vi "Motor_Ctrl.vi"(7 "Reset":bool, 8 "error in (no error)":errorcluster, 9 "TargetRPM(+/-120)":dbl format="%.2f", 10 "B/BL Motor":T1 items=["BLDC", "BDC"], 11 "Port":T2) -> (0 "error out":errorcluster, 1 "RPM/T Chart":cluster{"upper limit":dbl, "RPM":dbl}(graph), 2 "Rotations":dbl, 3 "RPM":dbl)   [LabVIEW 2019, in "Motor_Lib.lvlib"]
uses:
  Motor_Lib.lvlib
  PORT_ID.ctl
  MotorType.ctl
  <vilib>/myRIO/Instrument Drivers/Onboard IO/AO/typedefs/AO Reference.ctl
  <vilib>/myRIO/Common/Instrument Driver Framework/Utilities/typedefs/myRIO Generic Hardware Reference.ctl
  <vilib>/myRIO/Common/Instrument Driver Framework/Utilities/typedefs/Hardware Version Enum.ctl
  <vilib>/myRIO/Common/Instrument Driver Framework/Utilities/typedefs/myRIO v1.0 Reference.ctl
  <vilib>/myRIO/Common/Instrument Driver Framework/Utilities/typedefs/Generic FPGA Reference.ctl
  <vilib>/myRIO/Common/Instrument Driver Framework/myRIO v1.0/AO/typedefs/AO Channels List.ctl
  <vilib>/myRIO/Common/Instrument Driver Framework/myRIO v1.0/AO/typedefs/AO Channels Enum.ctl
  <vilib>/myRIO/Common/Instrument Driver Framework/Utilities/typedefs/Analog Scaling Constants List.ctl
  <vilib>/myRIO/Common/Instrument Driver Framework/Utilities/typedefs/Analog Scaling Constants.ctl
  <vilib>/userDefined/High Color/nirio_resource_hc.ctl
  <vilib>/myRIO/Instrument Drivers/Onboard IO/PWM/typedefs/PWM Reference.ctl
  <vilib>/myRIO/Common/Instrument Driver Framework/myRIO v1.0/PWM/typedefs/PWM Channels Enum.ctl
  <vilib>/myRIO/Instrument Drivers/Onboard IO/PWM/typedefs/PWM Configuration.ctl
  <vilib>/myRIO/Instrument Drivers/Onboard IO/DIO/typedefs/DIO Reference.ctl
  <vilib>/myRIO/Common/Instrument Driver Framework/myRIO v1.0/DIO/typedefs/DIO Channels List.ctl
  <vilib>/myRIO/Common/Instrument Driver Framework/myRIO v1.0/DIO/typedefs/DIO Channels Enum.ctl
  <vilib>/myRIO/Instrument Drivers/Onboard IO/PWM/vis/Set Duty Cycle and Frequency.vi
  <vilib>/myRIO/Common/Instrument Driver Framework/myRIO v1.0/PWM/vis/myRIO v1.1 Open PWM.vi
  <vilib>/myRIO/Common/Instrument Driver Framework/Utilities/vis/Is FPGA Ref Available.vi
  <vilib>/myRIO/Instrument Drivers/Onboard IO/DIO/vis/Write.vi
  <vilib>/myRIO/Common/Instrument Driver Framework/myRIO v1.0/DIO/vis/myRIO v1.1 Open DIO.vi
  <vilib>/myRIO/Instrument Drivers/Onboard IO/AO/vis/Write.vi
  <vilib>/myRIO/Common/Instrument Driver Framework/myRIO v1.0/AO/vis/myRIO v1.1 Open AO.vi
  <vilib>/myRIO/Common/Instrument Driver Framework/Utilities/vis/Validate Channels.vi
  <vilib>/myRIO/Common/Instrument Driver Framework/myRIO v1.0/PWM/vis/myRIO v1.0 Reserve PWM.vi
  <vilib>/myRIO/Common/Instrument Driver Framework/myRIO v1.0/DIO/vis/myRIO v1.0 Reserve DIO.vi
  <vilib>/myRIO/Common/Instrument Driver Framework/myRIO v1.0/AO/vis/myRIO v1.0 Reserve AO.vi
  <vilib>/myRIO/Common/Instrument Driver Framework/myRIO v1.0/PWM/vis/myRIO v1.0 Build MUX Configuration PWM.vi
  <vilib>/myRIO/Common/Instrument Driver Framework/myRIO v1.0/Resource Manager/vis/myRIO v1.0 Reserve Channel List.vi
  <vilib>/myRIO/Common/Instrument Driver Framework/myRIO v1.0/DIO/vis/myRIO v1.0 Build MUX Configuration DIO.vi
  <vilib>/myRIO/Common/Instrument Driver Framework/myRIO v1.0/AO/vis/myRIO v1.0 Build MUX Configuration AO.vi
  <vilib>/myRIO/Common/Instrument Driver Framework/myRIO v1.0/Resource Manager/vis/myRIO v1.0 Create Configuration List.vi
  <vilib>/myRIO/Common/Instrument Driver Framework/myRIO v1.0/Resource Manager/vis/myRIO v1.0 Reserve Channel.vi
  <vilib>/myRIO/Common/Instrument Driver Framework/myRIO v1.0/Resource Manager/vis/myRIO v1.0 Unreserve Channel.vi
  <vilib>/myRIO/Common/Instrument Driver Framework/myRIO v1.0/Resource Manager/vis/myRIO v1.0 Build Mutex Name.vi
  <vilib>/addons/control/pid/pid.llb/PID (DBL).vi
  <vilib>/Utility/VariantDataType/GetNumericInfo.vi
  <vilib>/Utility/error.llb/Error Cluster From Error Code.vi
  <vilib>/myRIO/Common/Instrument Driver Framework/myRIO v1.0/myRIO v1.1 Open.vi
  <vilib>/myRIO/Common/Instrument Driver Framework/myRIO v1.0/AO/vis/myRIO v1.0 Get Scaling Constants AO.vi
  <vilib>/myRIO/Common/Instrument Driver Framework/Utilities/vis/IO Manager.vi
  <vilib>/myRIO/Common/Instrument Driver Framework/Utilities/vis/Configuration Manager.vi
  <vilib>/myRIO/Common/Instrument Driver Framework/myRIO v1.0/myRIO v1.0 Close.vi
  <vilib>/myRIO/Common/Instrument Driver Framework/myRIO v1.0/AO/vis/myRIO v1.0 Write AO.vi
  <vilib>/myRIO/Common/Instrument Driver Framework/myRIO v1.0/Resource Manager/vis/myRIO v1.0 Configure IO.vi
  <vilib>/myRIO/Common/Instrument Driver Framework/myRIO v1.0/DIO/vis/myRIO v1.0 Write DIO.vi
  <vilib>/myRIO/Common/Instrument Driver Framework/myRIO v1.0/PWM/vis/myRIO v1.0 Write PWM.vi
  <vilib>/myRIO/Express VI/Onboard IO/AO/AO Express VI.xnode
  <vilib>/myRIO/Instrument Drivers/Onboard IO/AO/vis/myRIO AO Open.xnode
  <vilib>/myRIO/Express VI/Onboard IO/DO/DO Express VI.xnode
  <vilib>/myRIO/Instrument Drivers/Onboard IO/DIO/vis/myRIO DIO Open.xnode
  <vilib>/myRIO/Express VI/Onboard IO/PWM/PWM Express VI.xnode
  <vilib>/myRIO/Instrument Drivers/Onboard IO/PWM/vis/myRIO PWM Open.xnode
  <vilib>/myRIO/Instrument Drivers/Onboard IO/PWM/PWM.lvlib
  <vilib>/addons/control/pid/NI_PID_pid.lvlib
  <vilib>/myRIO/Instrument Drivers/Onboard IO/DIO/DIO.lvlib
  <vilib>/myRIO/Instrument Drivers/Onboard IO/AO/AO.lvlib
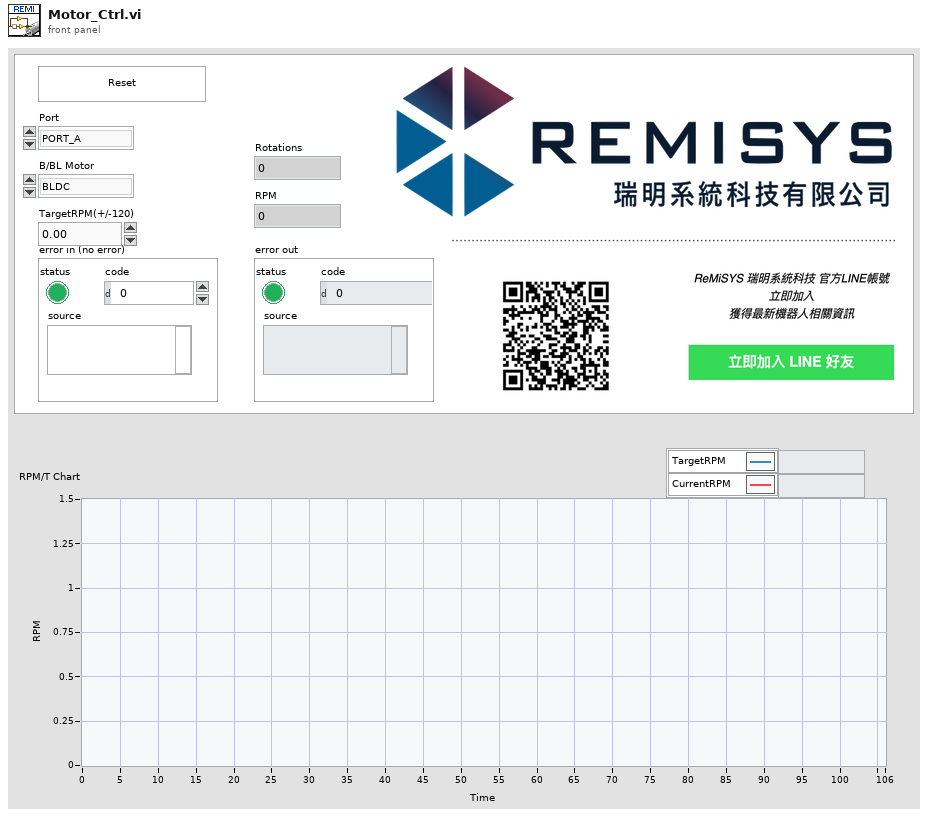
[diagram p1: front panel]
types:
  T1 = typedef "Motor_Lib.lvlib/MotorType.ctl" = u16
  T2 = typedef "Motor_Lib.lvlib/PORT_ID.ctl" = enum16{"PORT_A", "PORT_B"}
  T3 = cluster{"proportional gain (Kc)":dbl, "integral time (Ti, min)":dbl, "derivative time (Td, min)":dbl}
  T4 = typedef "AO.lvlib/AO Reference.ctl" = cluster{"myRIO Reference":T5, "AO Channel List":T9, "AO Scaling Constant List":T11}
  T5 = typedef "myRIO Generic Hardware Reference.ctl" = cluster{"myRIO Model":T6, "myRIO Hardware Reference":T7}
  T6 = typedef "Hardware Version Enum.ctl" = enum16{"Unknown", "myRIO-1900", "myRIO-1950", "roboRIO", "NI ELVIS RIO CM", "ELVIS III"}
  T7 = typedef "myRIO v1.0 Reference.ctl" = cluster{"Generic FPGA Reference":T8, "Allow multiple opens":bool}
  T8 = typedef "Generic FPGA Reference.ctl" = refnum<k20>
  T9 = typedef "AO Channels List.ctl" = T10[]
  T10 = typedef "AO Channels Enum.ctl" = enum16{"Not Connected", "AudioOut/Left", "AudioOut/Right", "C/AO0", "C/AO1", "A/AO0", "A/AO1", "B/AO0", "B/AO1"}
  T11 = typedef "Analog Scaling Constants List.ctl" = T12[]
  T12 = typedef "Analog Scaling Constants.ctl" = cluster{"LSB Weight (Volts)":dbl, "Offset (Volts)":dbl, "Signed?":bool}
  T13 = typedef "nirio_resource_hc.ctl" = tag
  T14 = typedef "DIO.lvlib/DIO Reference.ctl" = cluster{"myRIO Reference":T5, "DIO Channels List":T15}
  T15 = typedef "DIO Channels List.ctl" = T16[]
  T16 = typedef "DIO Channels Enum.ctl" = enum16{"Not Connected", "C/DIO0", "C/DIO1", "C/DIO2", "C/DIO3", "C/DIO4", "C/DIO5", "C/DIO6", "C/DIO7", "A/DIO0", "A/DIO1", "A/DIO2", "A/DIO3", "A/DIO4", "A/DIO5", "A/DIO6", "A/DIO7", "A/DIO8", "A/DIO9", "A/DIO10", "A/DIO11", "A/DIO12", "A/DIO13", "A/DIO14", "A/DIO15", "A/DIO16", "A/DIO17", "A/DIO18", "A/DIO19", "B/DIO0", "B/DIO1", "B/DIO2", "B/DIO3", "B/DIO4", "B/DIO5", "B/DIO6", "B/DIO7", "B/DIO8", "B/DIO9", "B/DIO10", "B/DIO11", "B/DIO12", "B/DIO13", "B/DIO14", "B/DIO15", "B/DIO16", "B/DIO17", "B/DIO18", "B/DIO19", "LED0", "LED1", "LED2", "LED3", "Button0", "DIO/DIO0", "DIO/DIO1", "DIO/DIO2", "DIO/DIO3", "DIO/DIO4", "DIO/DIO5", "DIO/DIO6", "DIO/DIO7", "DIO/DIO8", "DIO/DIO9", "SPI/CS0", "SPI/CS1", "SPI/CS2", "SPI/CS3", "LED RADIO (Green)", "LED RADIO (Red)", "LED COMM (Green)", "LED COMM (Red)", "LED MODE (Green)", "LED MODE (Red)"}
  T17 = typedef "PWM.lvlib/PWM Reference.ctl" = cluster{"myRIO Reference":T5, "PWM Channels Enum":T18, "PWM Configuration":T19}
  T18 = typedef "PWM Channels Enum.ctl" = enum16{"Not Connected", "C/PWM0", "C/PWM1", "A/PWM0", "A/PWM1", "A/PWM2", "A/PWM3", "A/PWM4", "A/PWM5", "A/PWM6", "A/PWM7", "A/PWM8", "A/PWM9", "A/PWM10", "A/PWM11", "A/PWM12", "A/PWM13", "A/PWM14", "A/PWM15", "A/PWM16", "A/PWM17", "A/PWM18", "A/PWM19", "B/PWM0", "B/PWM1", "B/PWM2", "B/PWM3", "B/PWM4", "B/PWM5", "B/PWM6", "B/PWM7", "B/PWM8", "B/PWM9", "B/PWM10", "B/PWM11", "B/PWM12", "B/PWM13", "B/PWM14", "B/PWM15", "B/PWM16", "B/PWM17", "B/PWM18", "B/PWM19", "PWM/PWM0", "PWM/PWM1", "PWM/PWM2", "PWM/PWM3", "PWM/PWM4", "PWM/PWM5", "PWM/PWM6", "PWM/PWM7", "PWM/PWM8", "PWM/PWM9"}
  T19 = typedef "PWM.lvlib/PWM Configuration.ctl" = cluster{"Frequency":dbl, "Duty Cycle":dbl}
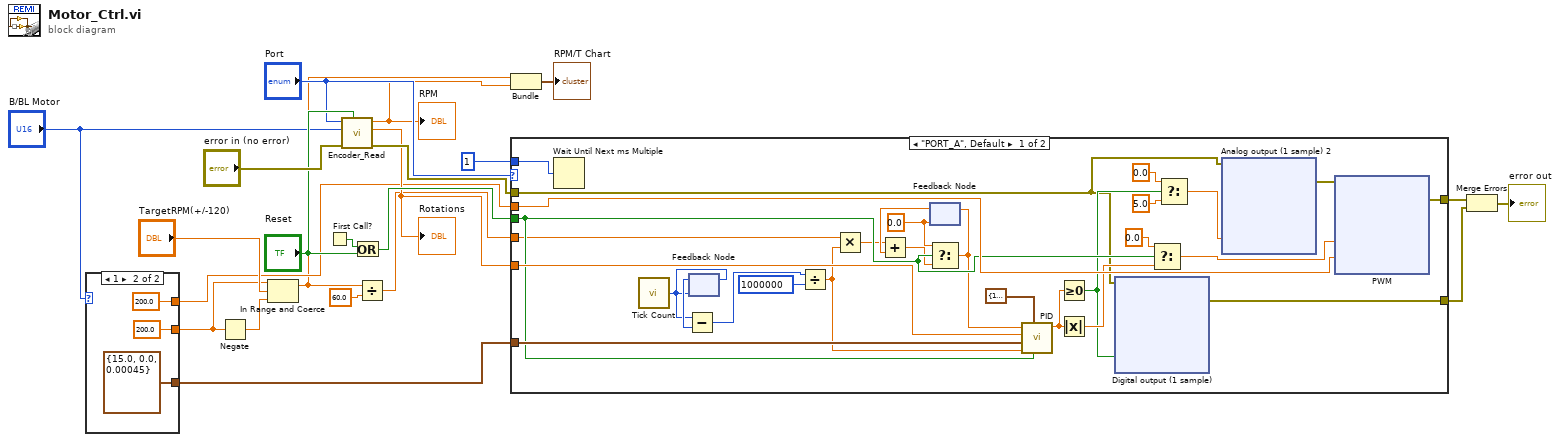
[diagram p0: block diagram]
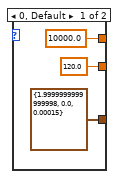
[diagram p2: hidden frame]
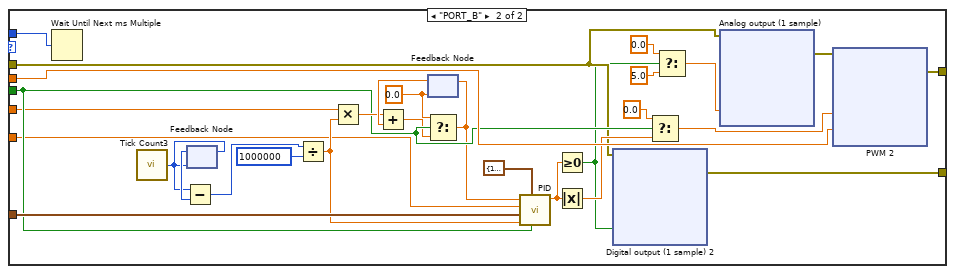
[diagram p3: hidden frame]
diagram:
  n1 = case shown="1" "B/BL Motor" {
    tunnel: [T3 {"proportional gain (Kc)"=1.9999999999999998, "integral time (Ti, min)"=0.0, "derivative time (Td, min)"=0.00015} ("PID gains") T3 {"proportional gain (Kc)"=15.0, "integral time (Ti, min)"=0.0, "derivative time (Td, min)"=0.00045} ("PID gains")] -> w17
    tunnel: [10000.0 ("Frequency [Hz]") 200.0 ("Frequency [Hz]")] -> w4
    tunnel: [120.0 ("upper limit") 200.0 ("upper limit")] -> w3
    frame 0, Default {
    }
    frame 1 {
    }
  }
  n2 = Negate(x=w3) -> (-x=w15:dbl)
  n3 = In Range and Coerce(upper limit=w3, x="TargetRPM(+/-120)", lower limit=w15) -> (coerced(x)=w2:dbl)  [unwired: 1 out]
  n4 = First Call?() -> (First Call?: T/F=w14:bool)
  n5 = call "Encoder_Read.vi"("Reset Counter"="Reset", "error in (no error)"="error in (no error)", "B/BL Motor"="B/BL Motor", "PORT"="Port") -> ("error out"=w22:errorcluster, "Rotations"=w6:dbl, "RPM"=w1:dbl)  [unwired: 5 in]
  "Rotations" <- w6
  "RPM" <- w1
  n6 = Or(x=w14, y="Reset") -> (x .or. y?=w12:bool)
  n7 = Divide(x=w2, y=60.0) -> (x/y=w5:dbl)
  n8 = Bundle("upper limit"=w2, "RPM"=w1) -> (→"RPM/T Chart":cluster{"upper limit":dbl, "RPM":dbl})  [unwired: 1 in]
  n9 = case shown="\"PORT_A\", Default" "Port" {
    tunnel: w4 -> [w57 w193]
    tunnel: w22 -> [w29 w170]
    tunnel: [w56 w192] -> w21
    tunnel: [w55 w168] -> w20
    tunnel: w17 -> [w49 w186]
    tunnel: w5 -> [w38 w166]
    tunnel: w6 -> [w48 w173]
    tunnel: w12 -> [w40 w176]
    tunnel: u32 1 ("millisecond multiple") -> [w31 w171]
    frame "PORT_A", Default {
      w39 = 0.0 ("setpoint")
      n10 = Wait Until Next ms Multiple(millisecond multiple=w31) -> ()  [unwired: 1 out]
      n11 = call "Tick Count"() -> ("Tick Count(uSec)"=w32:u32)
      n12 = feedback #1(w32) -> (w52:u32)
      n13 = Subtract(x=w32, y=w52) -> (x-y=w51:u32)
      n14 = feedback-in #1(w32) -> ()
      n15 = Divide(x=w51, y=u32 1000000) -> (x/y=w37:dbl)
      n16 = Multiply(x=w38, y=w37) -> (x*y=w35:dbl)
      n17 = feedback #2(w39) -> (w36:dbl)
      n18 = Add(x=w35, y=w36) -> (x+y=w34:dbl)
      n19 = Select(t=w39, s=w40, f=w34) -> (s? t:f=w33:dbl)
      n20 = feedback-in #2(w33) -> ()
      n21 = call-poly <vilib>:"PID.vi"("reinitialize? (F)"=w40, "output range"=cluster{"output high":dbl, "output low":dbl} {"output high"=1.0, "output low"=-1.0}, "dt (s)"=w37, "PID gains"=w49, "process variable"=w48, "setpoint"=w33) -> ("output"=w53:dbl)  [unwired: 4 in, 1 out]
      n22 = Greater Or Equal To 0?(x=w53) -> (x >= 0?=w30:bool)
      n23 = Absolute Value(x=w53) -> (abs(x)=w46:dbl)
      n24 = xnode "Digital output (1 sample)"("C/DIO1 (DIO1)"=w30, "error in (no error)"=w29) -> ("error out"=w55:errorcluster)
      n25 = Select(t=0.0, s=w40, f=w46) -> (s? t:f=w45:dbl)
      n26 = Select(t=0.0, s=w30, f=5.0) -> (s? t:f=w41:dbl)
      n27 = xnode "Analog output (1 sample) 2"("C/AO0 (AO0)"=w41, "error in (no error)"=w29) -> ("error out"=w44:errorcluster)
      n28 = xnode "PWM"("Duty Cycle"=w45, "Frequency [Hz]"=w57, "error in (no error)"=w44) -> ("error out"=w56:errorcluster)
    }
    frame "PORT_B" {
      w175 = 0.0 ("setpoint")
      n29 = Wait Until Next ms Multiple(millisecond multiple=w171) -> ()  [unwired: 1 out]
      n30 = call "Tick Count3"() -> ("Tick Count(uSec)"=w172:u32)
      n31 = feedback #3(w172) -> (w189:u32)
      n32 = Subtract(x=w172, y=w189) -> (x-y=w188:u32)
      n33 = feedback-in #3(w172) -> ()
      n34 = Divide(x=w188, y=u32 1000000) -> (x/y=w178:dbl)
      n35 = Multiply(x=w166, y=w178) -> (x*y=w177:dbl)
      n36 = feedback #4(w175) -> (w179:dbl)
      n37 = Add(x=w177, y=w179) -> (x+y=w174:dbl)
      n38 = Select(t=w175, s=w176, f=w174) -> (s? t:f=w165:dbl)
      n39 = feedback-in #4(w165) -> ()
      n40 = call-poly <vilib>:"PID.vi"("reinitialize? (F)"=w176, "output range"=cluster{"output high":dbl, "output low":dbl} {"output high"=1.0, "output low"=-1.0}, "dt (s)"=w178, "PID gains"=w186, "process variable"=w173, "setpoint"=w165) -> ("output"=w190:dbl)  [unwired: 4 in, 1 out]
      n41 = Greater Or Equal To 0?(x=w190) -> (x >= 0?=w167:bool)
      n42 = Absolute Value(x=w190) -> (abs(x)=w184:dbl)
      n43 = xnode "Digital output (1 sample) 2"("C/DIO5 (DIO5)"=w167, "error in (no error)"=w170) -> ("error out"=w168:errorcluster)
      n44 = Select(t=0.0, s=w176, f=w184) -> (s? t:f=w183:dbl)
      n45 = Select(t=0.0, s=w167, f=5.0) -> (s? t:f=w180:dbl)
      n46 = xnode "Analog output (1 sample)"("C/AO1 (AO1)"=w180, "error in (no error)"=w170) -> ("error out"=w169:errorcluster)
      n47 = xnode "PWM 2"("Duty Cycle"=w183, "Frequency [Hz]"=w193, "error in (no error)"=w169) -> ("error out"=w192:errorcluster)
    }
  }
  n48 = Merge Errors(w21, w20) -> (→"error out":errorcluster)
